vi "Close.vi"(8 "error in (no error)":errorcluster, 11 "SharedVariableWrapper in":refnum<class "SharedVariableWrapper.lvclass">) -> (0 "error out":errorcluster, 3 "SharedVariableWrapper out":refnum<class "SharedVariableWrapper.lvclass">)   [LabVIEW 2019, in "SharedVariableWrapper.lvclass"]
uses:
  SharedVariableWrapper.lvclass
  SharedVariableWrapper.lvclass/SharedVariableWrapper.ctl
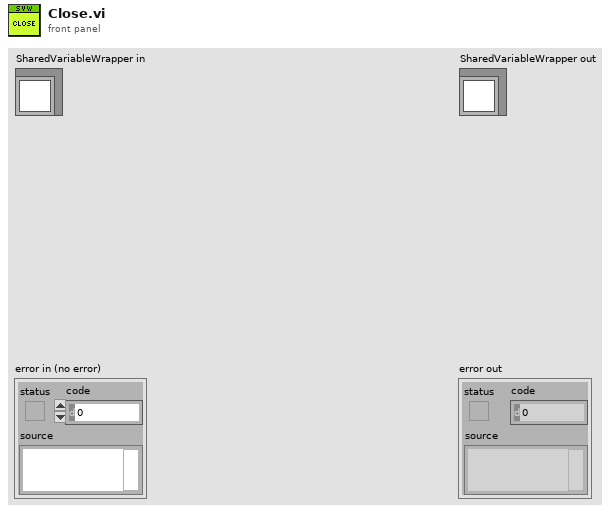
[diagram p1: front panel]
types:
  T1 = typedef "SharedVariableWrapper.lvclass/shared variable info.ctl" = cluster{"shared variable":refnum<k21>, "connected":bool, "Value":variant, "UpdateTime":timestamp}
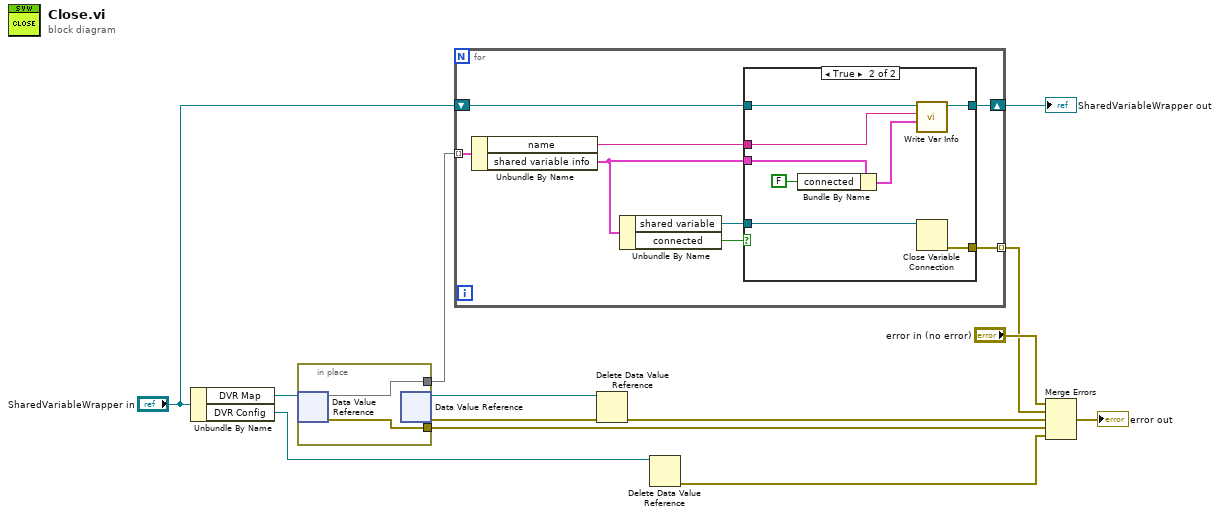
[diagram p0: block diagram]
diagram:
  n1 = Unbundle By Name("SharedVariableWrapper in") -> ("DVR Map"=w8:refnum<data-value>, "DVR Config"=w2:refnum<data-value>)
  n2 = in-place {
    in-place-border: [w15] -> w7
    in-place-border: [w14] -> w3
    n3 = in-place-dvr #1(w8) -> (w15:map{string, T1}, w14:errorcluster)
    n4 = in-place-dvr #1() -> (w6:refnum<data-value>, w5:errorcluster)  [unwired: 1 in]
  }
  n5 = for {
    tunnel: w7 -> [w23] mode=indexing
    shift-right: [w20] -> w10
    shift-left: "SharedVariableWrapper in" -> [w21]
    tunnel: [w19] -> w9 mode=indexing
    n6 = Unbundle By Name(w23) -> ("name"=w22:string, "shared variable info"=w16:T1)
    n7 = Unbundle By Name(w16) -> ("shared variable"=w18:refnum<k21>, "connected"=w17:bool)
    n8 = case shown="True" w17 {
      tunnel: w18 -> [_ w32]
      tunnel: w22 -> [_ w29]
      tunnel: w21 -> [w24 w31]
      tunnel: [w24 w30] -> w20
      tunnel: [_ w28] -> w19
      tunnel: w16 -> [_ w27]
      frame False {
      }
      frame True {
        n9 = Bundle By Name(cluster=w27, "connected"=FALSE) -> (w25:T1)
        n10 = call "Write Var Info.vi"("var info"=w25, "name"=w29, "SharedVariableWrapper in"=w31) -> ("SharedVariableWrapper out"=w30:refnum<class "SharedVariableWrapper.lvclass">)  [unwired: 7 in, 1 out]
        n11 = Close Variable Connection(11:w32) -> (0:w28:errorcluster)  [unwired: 1 in]
      }
    }
  }
  "SharedVariableWrapper out" <- w10
  n12 = Delete Data Value Reference(data value reference=w6, error in=w5) -> (error out=w4:errorcluster)  [unwired: 1 out]
  n13 = Delete Data Value Reference(data value reference=w2) -> (error out=w1:errorcluster)  [unwired: 1 in, 1 out]
  n14 = Merge Errors("error in (no error)", w9, w4, w3, w1) -> (→"error out":errorcluster)
